vi "Start absolute move.vi"(0 "Zaber":T1={"Serial port handle"="", "Axis"="", "Controller #"=0, "Min position"=0.0, "Max position"=0.0, "Min velocity"=0.0, "Max velocity"=0.0, "Firmware"="", "Device ID"=0, "Variable event"=refnum, "Variable ref"=refnum, "Resolution, usteps/step"=0, "Serial port semaphore"=refnum, "Joystick buttons"={"MinDir"=1, "MaxDir"=2, "MedSpeed"=5, "HighSpeed"=6}} {"Joystick buttons"."HighSpeed" min=1 max=25 step=1; "Joystick buttons"."MedSpeed" min=1 max=25 step=1; "Joystick buttons"."MaxDir" min=1 max=25 step=1; "Joystick buttons"."MinDir" min=1 max=25 step=1}, 2 "Position, mm":dbl, 5 "error in":errorcluster) -> (11 "Start time, ms":u32, 14 "Zaber out":T1={"Serial port handle"="", "Axis"="", "Controller #"=0, "Min position"=0.0, "Max position"=0.0, "Min velocity"=0.0, "Max velocity"=0.0, "Firmware"="", "Device ID"=0, "Variable event"=refnum, "Variable ref"=refnum, "Resolution, usteps/step"=0, "Serial port semaphore"=refnum, "Joystick buttons"={"MinDir"=1, "MaxDir"=2, "MedSpeed"=5, "HighSpeed"=6}} {"Joystick buttons"."HighSpeed" min=1 max=25 step=1; "Joystick buttons"."MedSpeed" min=1 max=25 step=1; "Joystick buttons"."MaxDir" min=1 max=25 step=1; "Joystick buttons"."MinDir" min=1 max=25 step=1}, 19 "error out":errorcluster)   [LabVIEW 2018]
uses:
  Zaber.ctl
  GenericDataEvent/GenericEvent.ctl
  ZaberVariables.ctl
  CommandZaber.ctl
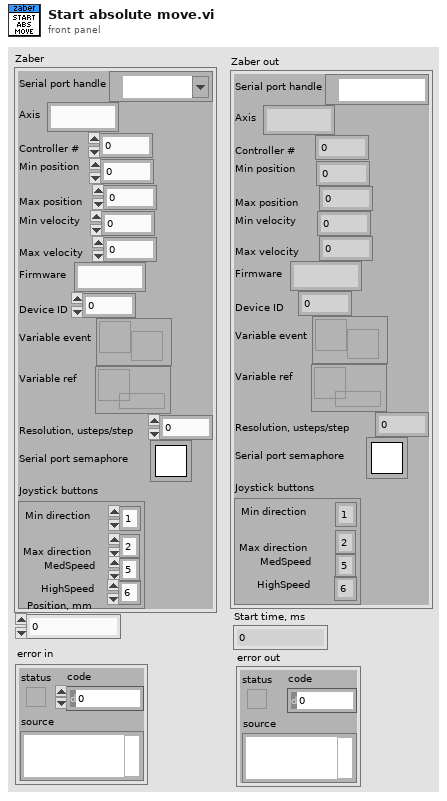
[diagram p1: front panel]
types:
  T1 = typedef "Zaber.ctl" = cluster{"Serial port handle":refnum<visa-resource-name>, "Axis":string, "Controller #":u8, "Min position":dbl, "Max position":dbl, "Min velocity":dbl, "Max velocity":dbl, "Firmware":string, "Device ID":i32, "Variable event":T2, "Variable ref":refnum<data-value>, "Resolution, usteps/step":i32, "Serial port semaphore":T3, "Joystick buttons":cluster{"MinDir":i32, "MaxDir":i32, "MedSpeed":i32, "HighSpeed":i32}}
  T2 = typedef "GenericEvent.ctl" = refnum<user-event>
  T3 = typedef "Semaphore RefNum" = refnum<k1>
  T4 = typedef "CommandZaber.ctl" = cluster{"Command":u8, "Data":i32}
  T5 = typedef "ZaberVariables.ctl" = cluster{"Position":i32, "Speed":i32, "Min soft position":dbl, "Max soft position":dbl, "Accelaration":i32}
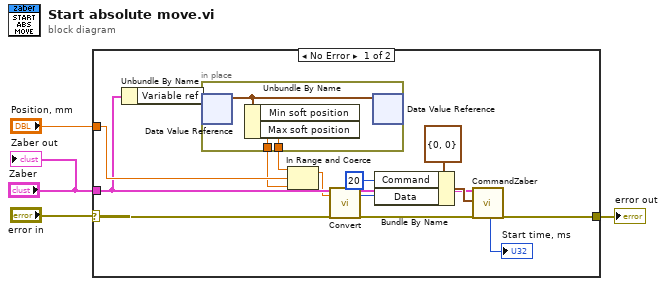
[diagram p0: block diagram]
diagram:
  n1 = case shown="No Error" "error in" {
    selector: "error in" -> [w14 w23]
    tunnel: [w8 w23] -> w3
    tunnel: "Zaber" -> [w12 _]
    tunnel: "Position, mm" -> [w16 _]
    frame No Error {
      n2 = Unbundle By Name(w12) -> ("Variable ref"=w7:refnum<data-value>)
      n3 = in-place {
        in-place-border: [w21] -> w6
        in-place-border: [w20] -> w5
        n4 = in-place-dvr #1(w7) -> (w22:T5)  [unwired: 1 out]
        n5 = Unbundle By Name(w22) -> ("Min soft position"=w21:dbl, "Max soft position"=w20:dbl)
        n6 = in-place-dvr #1(w22) -> ()  [unwired: 2 out]
      }
      n7 = In Range and Coerce(upper limit=w6, x=w16, lower limit=w5) -> (coerced(x)=w10:dbl)  [unwired: 1 out]
      n8 = call "Convert.vi"("Zaber"=w12, "Position, mm"=w10, "error in"=w14) -> ("Zaber out"=w11:T1, "Position, usteps"=w9:i32, "error out"=w13:errorcluster)  [unwired: 8 in, 6 out]
      n9 = Bundle By Name(cluster=T4 {"Command"=0, "Data"=0} ("Command"), "Command"=u8 20, "Data"=w9) -> (w19:T4)
      n10 = call "CommandZaber.vi"("Zaber"=w11, "Command"=w19, "error in"=w13) -> ("Command time, ms"=→"Start time, ms":u32, "error out"=w8:errorcluster)  [unwired: 13 in, 2 out]
    }
    frame Error {
    }
  }
  "error out" <- w3
  "Zaber out" <- "Zaber"
